vi "_Raise Context Menu Requested.vi"(4 "WebView2.lvlib:WebView2 Control.lvclass":refnum<class "WebView2 Control.lvclass">, 5 "Event Data":cluster{"sender":refnum<k24>, "e":refnum<k24>}, 6 "Control Ref":refnum<k24>, 7 "Event Common Data":T1) -> ()   [LabVIEW 2025, in "WebView2.lvlib" / "WebView2 Control.lvclass"]
uses:
  WebView2 Control.lvclass
  WebView2 Control.lvclass/WebView2 Control.ctl
  E:/Labview/LV 2023/PPL/PPL Builder/Libs/LV-WebView2/Source/Libs/Microsoft.Web.WebView2.Core.dll
  Libs/Microsoft.Web.WebView2.Core.dll
  System.Drawing
  Context Menu Requested Event Data.ctl
  WebView2 Event Filter Interface/WebView2 Event Filter Interface.lvclass
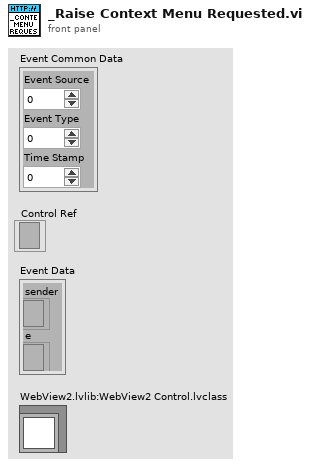
[diagram p1: front panel]
types:
  T1 = cluster{"Event Source":i32, "Event Type":u32, "Time Stamp":u32}
  T2 = typedef "WebView2.lvlib/WebView2 Control.lvclass/Context Menu Requested Event Data.ctl" = cluster{"ContextMenuTarget":refnum<k24>, "Location":refnum<k24>, "MenuItems":refnum<k24>}
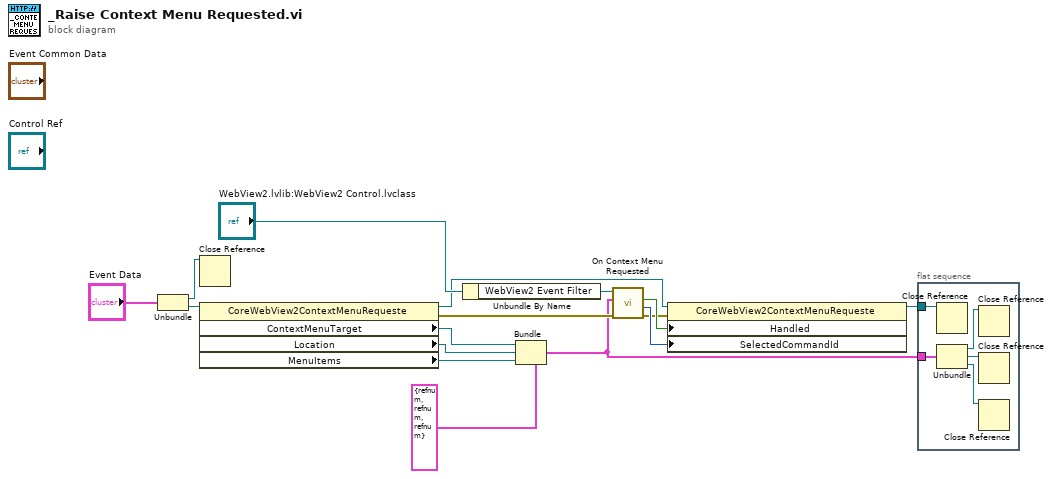
[diagram p0: block diagram]
diagram:
  n1 = Unbundle("Event Data") -> ("sender"=w14:refnum<k24>, "e"=w15:refnum<k24>)
  n2 = Close Reference(reference=w14) -> ()  [unwired: 1 in, 1 out]
  n3 = property class="CoreWebView2ContextMenuRequeste"(reference=w15) -> (reference out=w7:refnum<k24>, error out=w4:errorcluster, "ContextMenuTarget"=w13:refnum<k24>, "Location"=w11:refnum<k24>, "MenuItems"=w12:refnum<k24>)  [unwired: 1 in]
  n4 = Unbundle By Name("WebView2.lvlib:WebView2 Control.lvclass") -> ("WebView2 Event Filter"=w8:refnum<class "WebView2 Event Filter Interface.lvclass">)
  n5 = Bundle(cluster=T2 {"ContextMenuTarget"=refnum, "Location"=refnum, "MenuItems"=refnum}, "ContextMenuTarget"=w13, "Location"=w11, "MenuItems"=w12) -> (w1:T2)
  n6 = call-dynamic "On Context Menu Requested.vi"("error in (no error)"=w4, "Data"=w1, "WebView2 Event Filter Interface in"=w8) -> ("error out"=w3:errorcluster, "SelectedCommandId"=w5:i32, "Handled"=w6:bool)  [unwired: 6 in]
  n7 = property class="CoreWebView2ContextMenuRequeste"(reference=w7, error in=w3, "Handled"=w6, "SelectedCommandId"=w5) -> (reference out=w2:refnum<k24>)  [unwired: 1 out]
  n8 = flat-sequence {
    tunnel: w2 -> [w21]
    tunnel: w1 -> [w20]
    frame #0 {
      n9 = Close Reference(reference=w21) -> ()  [unwired: 1 in, 1 out]
      n10 = Unbundle(w20) -> ("ContextMenuTarget"=w19:refnum<k24>, "Location"=w18:refnum<k24>, "MenuItems"=w17:refnum<k24>)
      n11 = Close Reference(reference=w19) -> ()  [unwired: 1 in, 1 out]
      n12 = Close Reference(reference=w18) -> ()  [unwired: 1 in, 1 out]
      n13 = Close Reference(reference=w17) -> ()  [unwired: 1 in, 1 out]
    }
  }
